vi "FPGA Target.vi"() -> ()   [LabVIEW 2025]
uses:
  <vilib>/Platform/TimedLoop/XDataNode/wakeup.ctl
  <vilib>/Platform/TimedLoop/XDataNode/XDNodeRunTimeDep.lvlib
  <vilib>/Platform/TimedLoop/XDataNode/nitl_modes.ctl
  <vilib>/Platform/TimedLoop/XDataNode/timing_clust.ctl
  <vilib>/Platform/TimedLoop/XDataNode/XDataNode.xnode
  <vilib>/rvi/DataTransferAndStorage/Container/XNode/niFpgaContainer.xnode
  Templates/FPGA Wizard Templates.lvlib
  <vilib>/rvi/interface/RandomDataEmulation/nirviRandomDataFpgaReadWriteTemplate.vi
panel:
  out "Mod1.Monitor":bool[](array[boolean])
  in  "Accessory":bool
  in  "Key":bool
  in  "PWM Output 2":bool
  in  "PWM Output 1":bool
  in  "Crank":bool
  in  "Cam Exhaust":bool
  in  "Cam Intake":bool
  in  "Crank Temp":bool
  out "Mod3.Monitor":fxp<+/-,32,8>[](array[numeric])
  in  "Spare AO 2":fxp<+/-,32,8> format="%#_27g"
  in  "Spare AO 1":fxp<+/-,32,8> format="%#_27g"
  in  "Knock 1":fxp<+/-,32,8> format="%#_27g"
  in  "Crank VR":fxp<+/-,32,8> format="%#_27g"
  out "Pressure 3":fxp<+/-,32,8> format="%#_27g"
  out "Pressure 2":fxp<+/-,32,8> format="%#_27g"
  out "Pressure 1":fxp<+/-,32,8> format="%#_27g"
  out "Crank VR Loopback":fxp<+/-,32,8> format="%#_27g"
  out "Mod4.Monitor":fxp<+/-,20,5>[](array[numeric])
  out "Actual Analog Input Loop Period (usec)":u32
  out "Actual Analog Output Loop Period (usec)":u32
  out "Actual Digital Loop Period (usec)":u32
  out "Actual DMA Loop Period (usec)":u32
  in  "Analog Input Loop Timer (uSec)":u32=10
  in  "Digital Loop Timer (uSec)":u32=10
  in  "Analog Output Loop Timer (uSec)":u32=10
  in  "DMA.Enable":bool
  in  "DMA.MinimumSamples":u32=100000 caption="DMA Loop Timer (uSec)"
  out "DMA.Timeout":bool
  in  "DMA.Timeout.Reset":bool
  in  "DMA Loop Timer (uSec)":u32=10
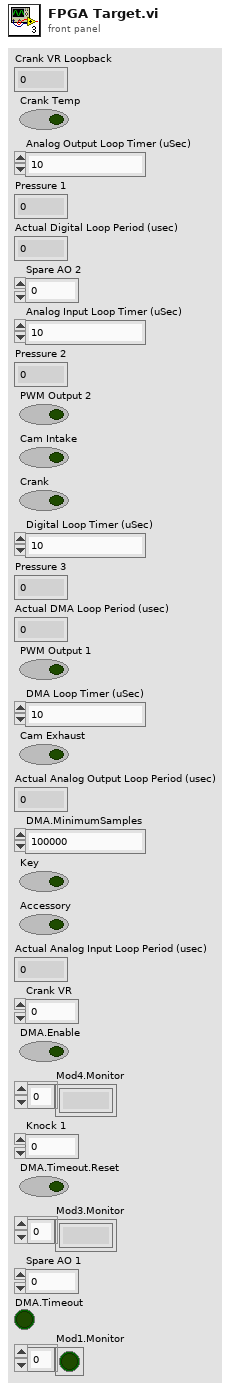
[diagram p1: front panel]
types:
  T1 = cluster{"DO 0":refnum<k21>, "DO 1":refnum<k21>, "DO 2":refnum<k21>, "DO 3":refnum<k21>, "DO 4":refnum<k21>, "DO 5":refnum<k21>, "DO 6":refnum<k21>, "DO 7":refnum<k21>}
  T2 = typedef "XDNodeRunTimeDep.lvlib/timing_clust.ctl" = cluster{"Expected End [f-1]":u64, "Actual End [f-1]":u64, "Finished Late? [f-1]":bool, "Expected End [i-1]":u64, "Actual End [i-1]":u64, "Finished Late? [i-1]":bool, "Expected Start [i]":u64, "Actual Start [i]":u64, "Expected Start [f]":u64, "Actual Start [f]":u64, "Source Name":string, "Structure Name":string, "Period":i64, "Deadline":i64, "Offset":i64, "Start":i64, "Priority":i32, "Timeout":i32, "Mode":T3, "Wakeup Reason":T4, "Error":errorcluster, "Source Type":string, "Secondary Source Type":string, "Global End Time":u64, "Global Start Time":u64, "Frame Duration":u64, "Iteration Duration":u64, "Assigned CPU":i32, "I/O Scan Engine Mode":u32}
  T3 = typedef "XDNodeRunTimeDep.lvlib/nitl_modes.ctl" = enum32{"No Change", "Process missed periods, maintain original phase", "Discard missed periods, maintain original phase", "Process missed periods, ignore original phase", "Discard missed periods, ignore original phase"}
  T4 = typedef "XDNodeRunTimeDep.lvlib/wakeup.ctl" = enum32{"Normal", "Aborted", "Asynchronous wakeup", "Timing source error", "Timed loop error", "Timeout"}
  T5 = cluster{"AO 0":refnum<k21>, "AO 1":refnum<k21>, "AO 2":refnum<k21>, "AO 3":refnum<k21>}
  T6 = cluster{"AI 0":refnum<k21>, "AI 1":refnum<k21>, "AI 2":refnum<k21>, "AI 3":refnum<k21>}
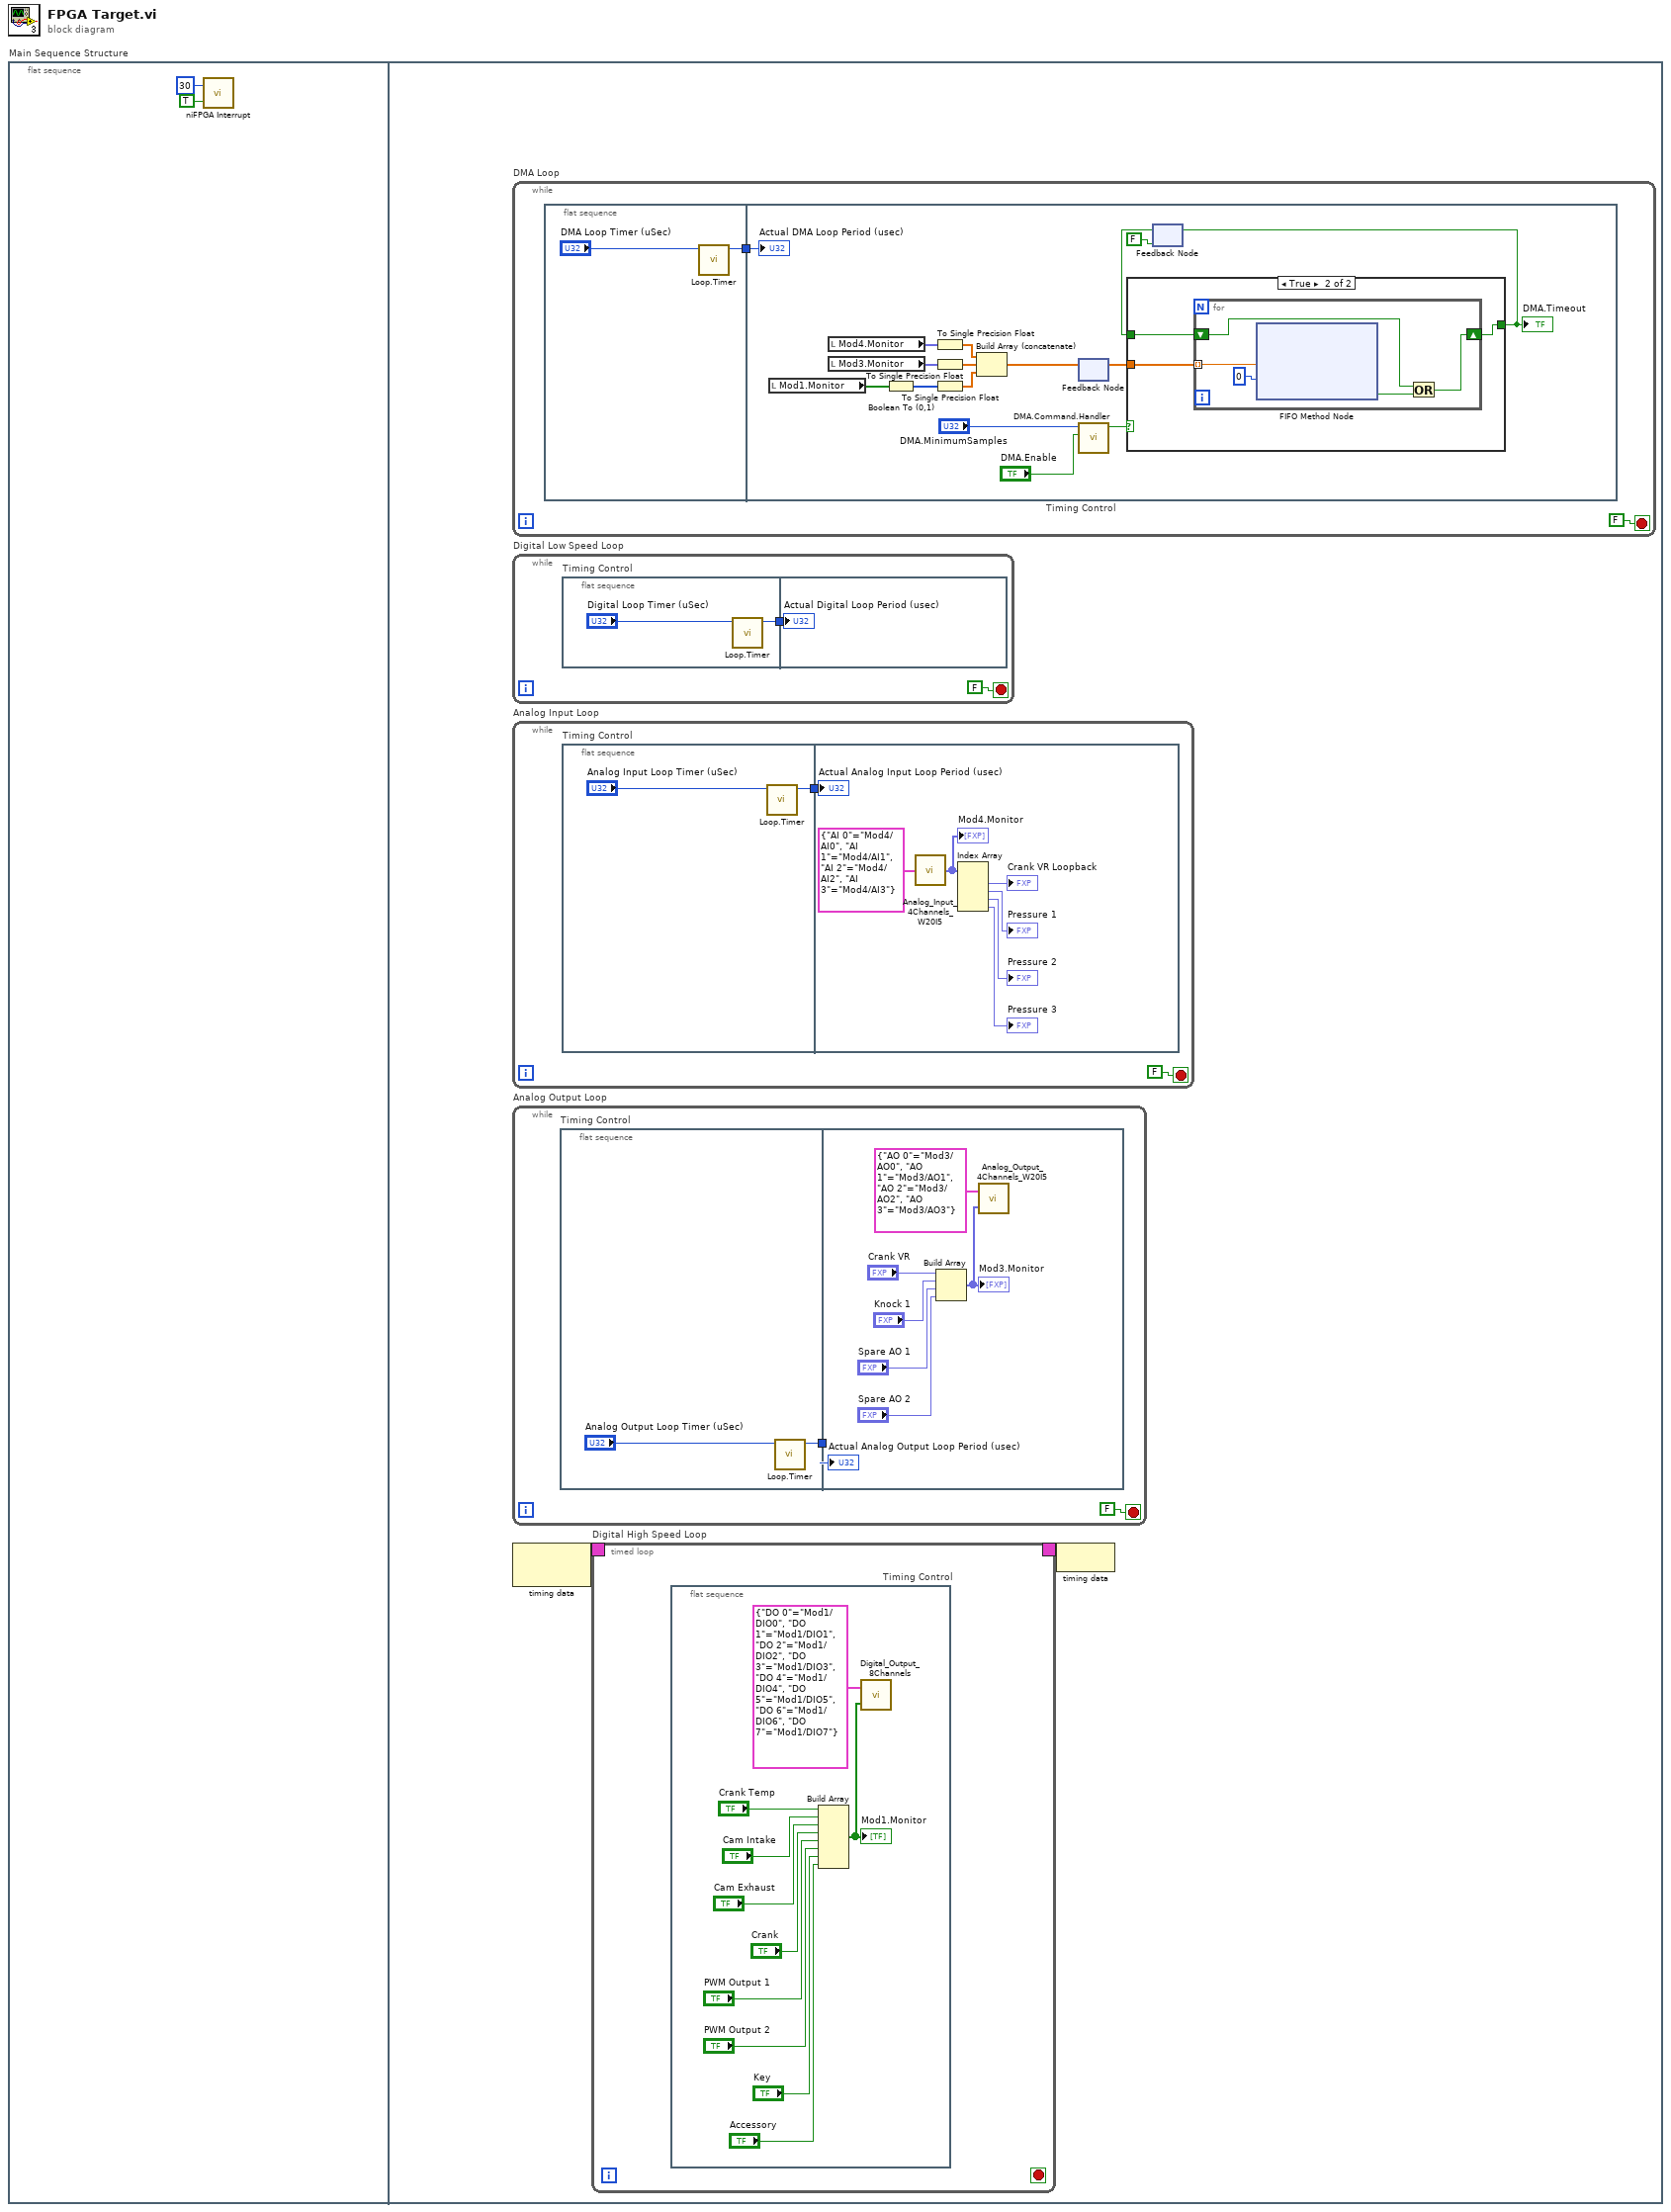
[diagram p0: block diagram]
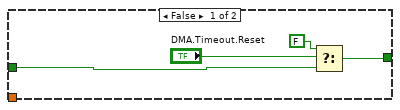
[diagram p2: hidden frame]
diagram:
  n1 = flat-sequence "Main Sequence Structure" {
    frame #0 {
      n2 = call <vilib>:"niFPGA Interrupt.vi"("Wait Until Cleared (F)"=TRUE, "IRQ Number (0)"=u8 30) -> ()  [unwired: 1 in]
    }
    frame #1 {
      # "FPGA Addon Code"
      n3 = while "DMA Loop" {
        stop <- FALSE stop-if-true
        n4 = flat-sequence "Timing Control" {
          tunnel: [w21] -> w19
          tunnel: w19 -> [w30]
          frame #0 {
            n5 = call "Loop.Timer.vi"("Loop Timer (uSec)"="DMA Loop Timer (uSec)") -> ("Actual Loop Period (usec)"=w21:u32)  [unwired: 10 in]
          }
          frame #1 {
            n6 = local read "Mod1.Monitor"() -> (w27:bool[])
            n7 = local read "Mod4.Monitor"() -> (w29:fxp<+/-,20,5>[])
            n8 = local read "Mod3.Monitor"() -> (w28:fxp<+/-,32,8>[])
            n9 = Boolean To (0,1)(Boolean=w27) -> (0, 1=w26:i16[])
            n10 = To Single Precision Float(number=w29) -> (single precision float=w25:sgl[])
            n11 = To Single Precision Float(number=w28) -> (single precision float=w24:sgl[])
            n12 = To Single Precision Float(number=w26) -> (single precision float=w23:sgl[])
            n13 = Build Array (concatenate) "Build Array"(w25, w24, w23) -> (w36:sgl[])
            n14 = feedback #1() -> (w35:sgl[])  [unwired: 1 in]
            n15 = feedback-in #1(w36) -> ()
            n16 = call "DMA.Command.Handler.vi"("DMA.Enable"="DMA.Enable", "DMA.MinimumSamples"="DMA.MinimumSamples") -> ("Transfer"=w32:bool)  [unwired: 9 in]
            n17 = feedback #2(FALSE ("t")) -> (w31:bool)
            n18 = case shown="True" w32 {
              tunnel: w35 -> [_ w45]
              tunnel: w31 -> [w40 w44]
              tunnel: [w39 w43] -> w34
              frame False {
                n19 = Select(t=FALSE, s="DMA.Timeout.Reset", f=w40) -> (s? t:f=w39:bool)
              }
              frame True {
                n20 = for {
                  shift-right: [w48] -> w43
                  shift-left: w44 -> [w47]
                  tunnel: w45 -> [w46] mode=indexing
                  n21 = xnode ("FIFO Method Node")("Element"=w46, "Timeout"=0) -> ("Timed Out?"=w49:bool)  [unwired: 1 in, 1 out]
                  n22 = Or(x=w47, y=w49) -> (x .or. y?=w48:bool)
                }
              }
            }
            "DMA.Timeout" <- w34
            n23 = feedback-in #2(w34) -> ()
            "Actual DMA Loop Period (usec)" <- w30
          }
        }
      }
      n24 = while "Digital Low Speed Loop" {
        stop <- FALSE stop-if-true
        n25 = flat-sequence "Timing Control" {
          tunnel: [w75] -> w73
          tunnel: w73 -> [w77]
          frame #0 {
            n26 = call "Loop.Timer.vi"("Loop Timer (uSec)"="Digital Loop Timer (uSec)") -> ("Actual Loop Period (usec)"=w75:u32)  [unwired: 10 in]
          }
          frame #1 {
            "Actual Digital Loop Period (usec)" <- w77
          }
        }
      }
      n27 = while "Analog Input Loop" {
        stop <- FALSE stop-if-true
        n28 = flat-sequence "Timing Control" {
          tunnel: [w64] -> w62
          tunnel: w62 -> [w72]
          frame #0 {
            n29 = call "Loop.Timer.vi"("Loop Timer (uSec)"="Analog Input Loop Timer (uSec)") -> ("Actual Loop Period (usec)"=w64:u32)  [unwired: 10 in]
          }
          frame #1 {
            n30 = call "Analog_Input_4Channels_W20I5.vi"("IO"=T6 {"AI 0"="Mod4/AI0", "AI 1"="Mod4/AI1", "AI 2"="Mod4/AI2", "AI 3"="Mod4/AI3"}) -> ("Values"=w70:fxp<+/-,20,5>[])
            "Mod4.Monitor" <- w70
            n31 = Index Array(array=w70) -> (element #1=→"Crank VR Loopback":fxp<+/-,20,5>, element #2=→"Pressure 1":fxp<+/-,20,5>, element #3=→"Pressure 2":fxp<+/-,20,5>, element #4=→"Pressure 3":fxp<+/-,20,5>)  [unwired: 4 in]
            "Actual Analog Input Loop Period (usec)" <- w72
          }
        }
      }
      n32 = while "Analog Output Loop" {
        stop <- FALSE stop-if-true
        n33 = flat-sequence "Timing Control" {
          tunnel: [w53] -> w51
          tunnel: w51 -> [w61]
          frame #0 {
            n34 = call "Loop.Timer.vi"("Loop Timer (uSec)"="Analog Output Loop Timer (uSec)") -> ("Actual Loop Period (usec)"=w53:u32)  [unwired: 10 in]
          }
          frame #1 {
            n35 = Build Array("Crank VR", "Knock 1", "Spare AO 1", "Spare AO 2") -> (w55:fxp<+/-,32,8>[])
            "Mod3.Monitor" <- w55
            n36 = call "Analog_Output_4Channels_W20I5.vi"("Values"=w55, "IO"=T5 {"AO 0"="Mod3/AO0", "AO 1"="Mod3/AO1", "AO 2"="Mod3/AO2", "AO 3"="Mod3/AO3"}) -> ()  [unwired: 1 in]
            "Actual Analog Output Loop Period (usec)" <- w61
          }
        }
      }
      n37 = node-c288() -> (w4:T2)  [unwired: 1 in]
      n38 = timed-loop "Digital High Speed Loop" {
        timing: w4 -> [_]
        timing-out: [_] -> w3
        stop <- _ stop-if-true
        n39 = flat-sequence "Timing Control" {
          frame #0 {
            n40 = Build Array("Crank Temp", "Cam Intake", "Cam Exhaust", "Crank", "PWM Output 1", "PWM Output 2", "Key", "Accessory") -> (w5:bool[])
            "Mod1.Monitor" <- w5
            n41 = call "Digital_Output_8Channels.vi"("States"=w5, "IO"=T1 {"DO 0"="Mod1/DIO0", "DO 1"="Mod1/DIO1", "DO 2"="Mod1/DIO2", "DO 3"="Mod1/DIO3", "DO 4"="Mod1/DIO4", "DO 5"="Mod1/DIO5", "DO 6"="Mod1/DIO6", "DO 7"="Mod1/DIO7"}) -> ()  [unwired: 1 in]
          }
        }
      }
      n42 = node-c288 ("Output Node")(w3) -> ()
    }
  }
